vi "Get Event Timing Measurements - Multi FPGA.vi"(7 "return not-added measurements (T)":bool=TRUE, 8 "error in (no error)":errorcluster, 10 "RIO Address":string, 11 "Item Ref in":T1 format="%.0x") -> (0 "error out":errorcluster, 1 "measurements refs":T1[](array[typedef]) format="%.0x", 2 "measurements":T2[](array[typedef]), 3 "Item Ref out":T1 format="%.0x", 5 "not present indexes":i32[](array[numeric]))   [LabVIEW 2017, in "Engine Simulation Toolkit System Explorer.lvlib"]
uses:
  Engine Simulation Toolkit System Explorer.lvlib
  Event Timing Measurement.ctl
  Polarity.ctl
  <vilib>/NI Veristand/Custom Device API/Custom Device Item Ref.ctl
  Shared/Properties.vi
  <vilib>/NI Veristand/Custom Device API/Get Item Property (String).vi
  Shared/Constants and GUIDs.vi
  <vilib>/NI Veristand/Custom Device API/Get Item Property (U16).vi
  Shared/Engine Simulation Toolkit Shared.lvlib
  <vilib>/NI Veristand/Custom Device API/Custom Device API.lvlib
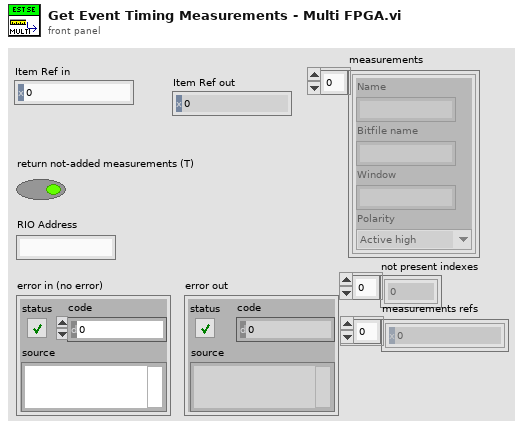
[diagram p1: front panel]
types:
  T1 = typedef "Custom Device API.lvlib/Custom Device Item Ref.ctl" = u64
  T2 = typedef "Engine Simulation Toolkit System Explorer.lvlib/Event Timing Measurement.ctl" = cluster{"Name":string, "Bitfile name":string, "Window":string, "Polarity":T3}
  T3 = typedef "Engine Simulation Toolkit System Explorer.lvlib/Polarity.ctl" = enum16{"Active low", "Active high"}
  T4 = typedef "Custom Device API.lvlib/Custom Device Item Info.ctl" = cluster{"Name":string, "Is Channel":bool, "GUID":string, "Is Waveform":bool}
  T5 = cluster{"ip list property name":string, string[]}[]
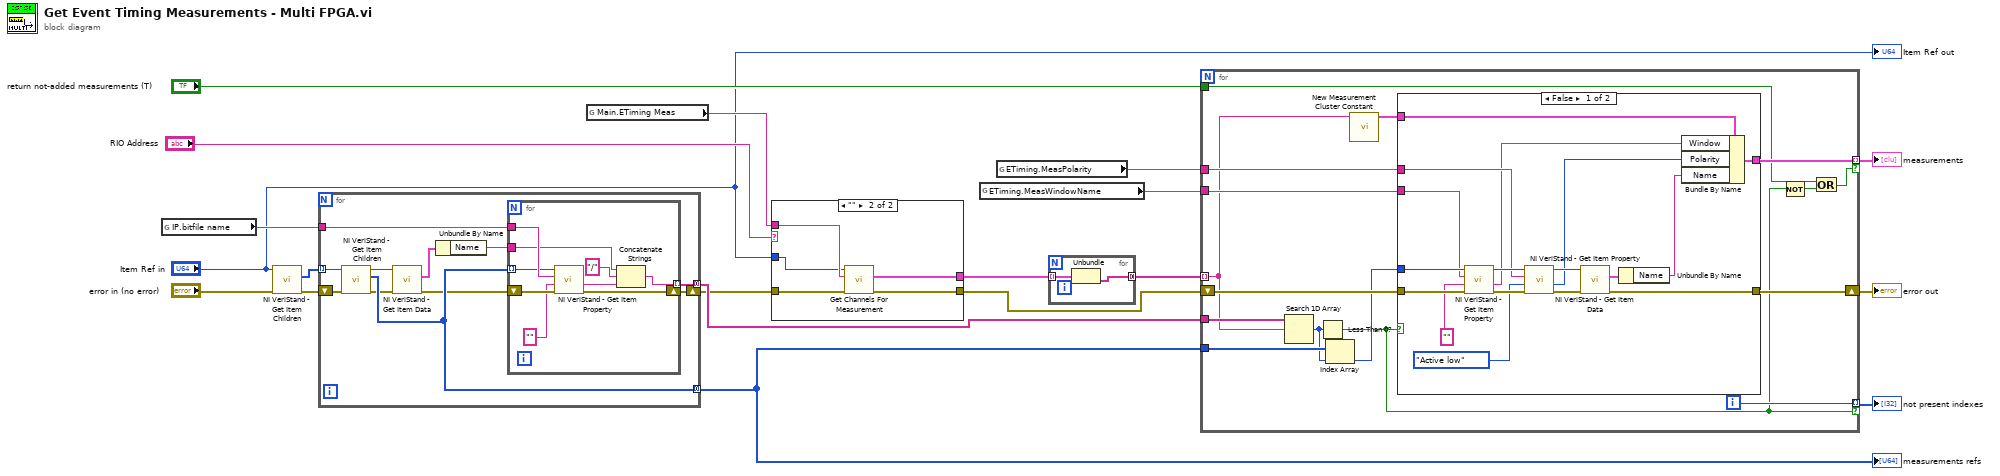
[diagram p0: block diagram]
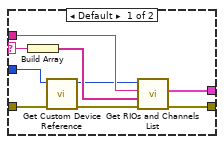
[diagram p2: hidden frame]
diagram:
  n1 = global read "Properties.vi" "IP.bitfile name"() -> (w14:string)
  n2 = call <vilib>:"NI VeriStand - Get Item Children.vi"("error in (no error)"="error in (no error)", "Item Ref in"="Item Ref in") -> ("error out"=w10:errorcluster, "Child Refs"=w9:T1[])  [unwired: 6 in, 2 out]
  n3 = for {
    tunnel: w14 -> [w30]
    tunnel: [w29] -> w7 mode=concatenating
    tunnel: [w28] -> w13 mode=concatenating
    tunnel: w9 -> [w26] mode=indexing
    shift-right: [w27] -> w2
    shift-left: w10 -> [w25]
    n4 = call <vilib>:"NI VeriStand - Get Item Children.vi"("error in (no error)"=w25, "Item Ref in"=w26) -> ("error out"=w23:errorcluster, "Child Refs"=w28:T1[], "Item Ref out"=w21:T1)  [unwired: 6 in, 1 out]
    n5 = call <vilib>:"NI VeriStand - Get Item Data.vi"("error in (no error)"=w23, "Item Ref in"=w21) -> ("error out"=w22:errorcluster, "Item Info"=w20:T4)  [unwired: 6 in, 2 out]
    n6 = Unbundle By Name(w20) -> ("Name"=w24:string)
    n7 = for {
      shift-right: [w37] -> w27
      shift-left: w22 -> [w39]
      tunnel: w28 -> [w31] mode=indexing
      tunnel: w30 -> [w38]
      tunnel: [w32] -> w29 mode=indexing
      tunnel: w24 -> [w33]
      n8 = call-poly <vilib>:"NI VeriStand - Get Item Property.vi"("error in (no error)"=w39, "Default Value"="", "Property Name"=w38, "Item Ref in"=w31) -> ("error out"=w37:errorcluster, "Value"=w35:string)  [unwired: 4 in, 2 out]
      n9 = Concatenate Strings(w33, "/" ("string"), w35) -> (w32:string)
    }
  }
  "measurements refs" <- w13
  n10 = global read "Properties.vi" "Main.ETiming Meas"() -> (w5:string)
  n11 = case shown="\"\"" "RIO Address" {
    selector: "RIO Address" -> [w48 _]
    tunnel: w2 -> [w45 w53]
    tunnel: w5 -> [w47 w50]
    tunnel: [w42 w52] -> w4
    tunnel: [w41 w51] -> w3
    tunnel: "Item Ref in" -> [w40 w49]
    frame Default {
      n12 = Build Array(w48) -> (w46:string[])
      n13 = call "Get Custom Device Reference.vi"("error in (no error)"=w45, "Item Ref in"=w40) -> ("error out"=w44:errorcluster, "Item Ref out"=w43:T1)  [unwired: 7 in, 1 out]
      n14 = call "Get RIOs and Channels List.vi"("error in (no error)"=w44, "rio names"=w46, "ip list property name"=w47, "Item Ref in"=w43) -> ("error out"=w42:errorcluster, "rios and channels"=w41:T5)  [unwired: 5 in, 1 out]
    }
    frame "" {
      n15 = call "Get Channels For Measurement.vi"("error in (no error)"=w53, "property name"=w50, "Node Ptr in"=w49) -> ("error out"=w52:errorcluster, "rios and channels"=w51:T5)  [unwired: 6 in, 1 out]
    }
  }
  n16 = global read "Properties.vi" "ETiming.MeasWindowName"() -> (w17:string)
  n17 = global read "Properties.vi" "ETiming.MeasPolarity"() -> (w16:string)
  n18 = for {
    tunnel: w3 -> [w55] mode=indexing
    tunnel: [w54] -> w11 mode=concatenating
    n19 = Unbundle(w55) -> (w54:string[])  [unwired: 1 out]
  }
  n20 = for {
    tunnel: [w61] -> w19 mode=indexing if=w59
    shift-right: [w69] -> w18
    shift-left: w4 -> [w67]
    tunnel: w11 -> [w56] mode=indexing
    tunnel: w17 -> [w71]
    tunnel: w16 -> [w70]
    tunnel: [w68] -> w15 mode=indexing if=w60
    tunnel: w7 -> [w66]
    tunnel: w13 -> [w65]
    tunnel: "return not-added measurements (T)" -> [w58]
    i -> [w68]
    n21 = Search 1D Array(1D array=w66, element=w56) -> (index of element=w64:i32)  [unwired: 1 in]
    n22 = Less Than 0?(x=w64) -> (x < 0?=w60:bool)
    n23 = Index Array(array=w65, index=w64) -> (element=w63:T1)
    n24 = call "New Measurement Cluster Constant.vi"("Bitfile name"=w56) -> ("Measurement"=w62:T2)  [unwired: 10 in]
    n25 = case shown="False" w60 {
      tunnel: w67 -> [w88 w90]
      tunnel: w63 -> [w87 _]
      tunnel: w71 -> [w86 _]
      tunnel: w70 -> [w83 _]
      tunnel: [w81 w90] -> w69
      tunnel: w62 -> [w76 w89]
      tunnel: [w72 w89] -> w61
      frame False {
        n26 = call-poly <vilib>:"NI VeriStand - Get Item Property.vi"("error in (no error)"=w88, "Default Value"="", "Property Name"=w86, "Item Ref in"=w87) -> ("error out"=w85:errorcluster, "Value"=w75:string, "Item Ref out"=w84:T1)  [unwired: 4 in, 1 out]
        n27 = call-poly <vilib>:"NI VeriStand - Get Item Property.vi"("error in (no error)"=w85, "Default Value"=Polarity."Active low" ("Polarity"), "Property Name"=w83, "Item Ref in"=w84) -> ("error out"=w82:errorcluster, "Value"=w74:u16, "Item Ref out"=w77:T1)  [unwired: 4 in, 1 out]
        n28 = call <vilib>:"NI VeriStand - Get Item Data.vi"("error in (no error)"=w82, "Item Ref in"=w77) -> ("error out"=w81:errorcluster, "Item Info"=w80:T4)  [unwired: 6 in, 2 out]
        n29 = Unbundle By Name(w80) -> ("Name"=w73:string)
        n30 = Bundle By Name(cluster=w76, "Window"=w75, "Polarity"=w74, "Name"=w73) -> (w72:T2)
      }
      frame True {
      }
    }
    n31 = Not(x=w60) -> (.not. x?=w57:bool)
    n32 = Or(x=w58, y=w57) -> (x .or. y?=w59:bool)
  }
  "error out" <- w18
  "measurements" <- w19
  "not present indexes" <- w15
  "Item Ref out" <- "Item Ref in"
